vi "CameraAngleMath.vi"(11 "TargetXCenter":dbl) -> (3 "TargetAngle":dbl)   [LabVIEW 2016]
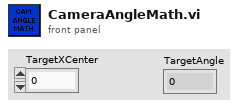
[diagram p1: front panel]
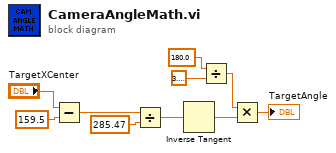
[diagram p0: block diagram]
diagram:
  n1 = Subtract(x="TargetXCenter", y=159.5) -> (x-y=w9:dbl)
  n2 = Divide(x=w9, y=285.47) -> (x/y=w7:dbl)
  n3 = Inverse Tangent(1:w7) -> (0:w6:dbl)
  n4 = Divide(x=180.0, y=3.141592653589793) -> (x/y=w3:dbl)
  n5 = Multiply(x=w3, y=w6) -> (x*y=→"TargetAngle":dbl)
